vi "BRig_dataExp_LaserSwitch.vi"() -> (2 "output_LaserSwitch":i32)   [LabVIEW 2014]
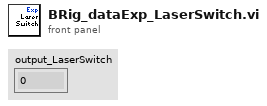
[diagram p1: front panel]
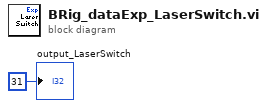
[diagram p0: block diagram]
diagram:
  "output_LaserSwitch" <- 31 ("output_iBlock")
